vi "PV ActiveLine - Ethernet MAC Address.vi"(3 "Fehler (Eingang)":errorcluster, 5 "Referenz in":refnum<visa-resource-name>) -> (0 "Cluster (Ausgang)":errorcluster caption="Fehler (Ausgang)", 1 "MAC address":string, 2 "Referenz out":refnum<visa-resource-name>)   [LabVIEW 2013, in "PV ActiveLine.lvlib"]
doc: "MAC - Ethernet MAC Address\n\nTransmit: MAC\nReceive: aa-aa-aa-aa-aa-aa\n\nEthernet MAC address of the TPG 36x:\n00-A0-41-xx-xx-xx"
uses:
  <instrlib>/PV ActiveLine/PV ActiveLine.lvlib
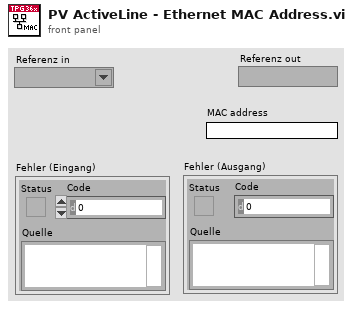
[diagram p1: front panel]
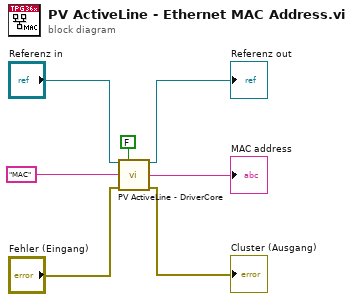
[diagram p0: block diagram]
diagram:
  n1 = call <instrlib>:"PV ActiveLine - DriverCore.vi"("Referenz in"="Referenz in", "Write/Read"=FALSE, "Command"="MAC", "Fehler (Eingang)"="Fehler (Eingang)") -> ("Referenz out"=→"Referenz out":refnum<visa-resource-name>, "String Out"=→"MAC address":string, "Cluster (Ausgang)"=→"Cluster (Ausgang)":errorcluster)  [unwired: 9 in]
